vi "Extract Data.vi"(8 "error in (no error)":errorcluster caption="entrée d'erreur (pas d'erreur)", 11 "Parsing Data RADIO_ERP1 en entrée":refnum<class "Parsing Data RADIO_ERP1_D5.lvclass">) -> (0 "error out":errorcluster caption="sortie d'erreur", 3 "Parsing Data RADIO_ERP1 en sortie":refnum<class "Parsing Data RADIO_ERP1_D5.lvclass">)   [LabVIEW 2020, in "Library Instrument & Equipement.lvlib" / "Library UART.lvlib" / "Parsing Data RADIO_ERP1_D5.lvclass"]
uses:
  Parsing Data RADIO_ERP1_D5.lvclass
  C:/Users/ngarcin/OneDrive - Altyor/Standard TB/Class/UART/UART Enocean/Parsing Data Enocean (Default)/Parsing Data Enocean (Default).lvclass
  Parsing Data RADIO_ERP1_D5.lvclass/Parsing Data RADIO_ERP1_D5.ctl
  Commun VI/Library Commun.lvlib
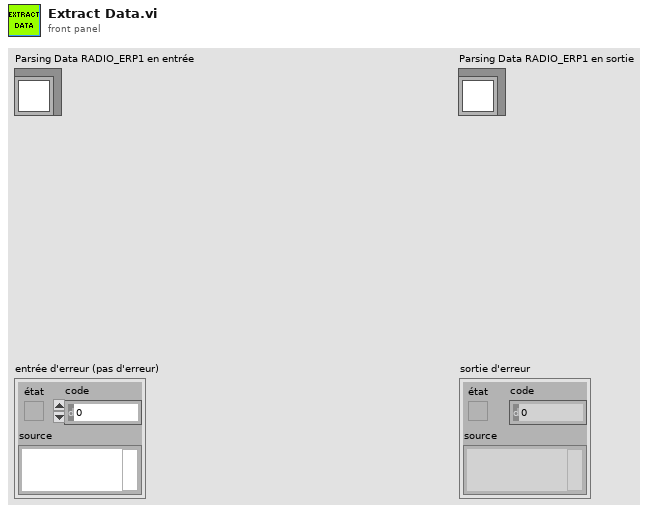
[diagram p1: front panel]
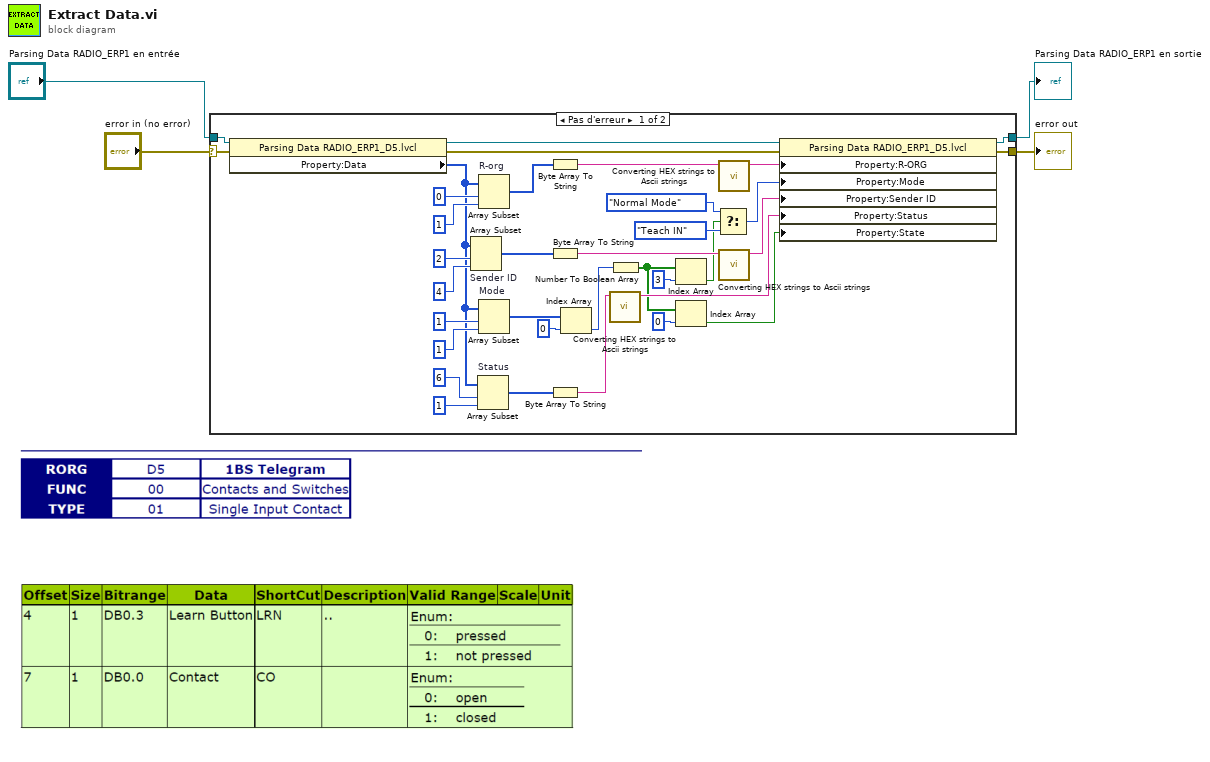
[diagram p0: block diagram]
diagram:
  n1 = case shown="Pas d'erreur" "error in (no error)" {
    selector: "error in (no error)" -> [w25 w41]
    tunnel: [w24 w41] -> w4
    tunnel: [w26 w40] -> w3
    tunnel: "Parsing Data RADIO_ERP1 en entrée" -> [w27 w40]
    frame No Error {
      n2 = property class="Parsing Data RADIO_ERP1_D5.lvcl"(reference=w27, error in=w25) -> (reference out=w39:refnum<class "Parsing Data RADIO_ERP1_D5.lvclass">, error out=w28:errorcluster, "Property:Data"=w15:u8[])
      n3 = Array Subset "Sender ID"(array=w15, index=2 ("indice"), length=4 ("longueur")) -> (w34:u8[])
      n4 = Array Subset "Status"(array=w15, index=6 ("indice"), length=1 ("indice")) -> (w29:u8[])
      n5 = Array Subset "R-org"(array=w15, index=0 ("indice"), length=1 ("longueur")) -> (w37:u8[])
      n6 = Array Subset "Mode"(array=w15, index=1 ("indice"), length=1 ("longueur")) -> (w13:u8[])
      n7 = Byte Array To String(unsigned byte array=w37) -> (string=w36:string)
      n8 = Byte Array To String(unsigned byte array=w34) -> (string=w33:string)
      n9 = Byte Array To String(unsigned byte array=w29) -> (string=w31:string)
      n10 = Index Array(array=w13, index=0 ("indice")) -> (element=w12:u8)
      n11 = call "Converting HEX strings to Ascii strings.vi"("chaîne IN"=w31) -> ("Chaîne OUT"=w30:string)  [unwired: 9 in, 1 out]
      n12 = Number To Boolean Array(number=w12) -> (Boolean array=w10:bool[])
      n13 = Index Array(array=w10, index=3 ("indice")) -> (element=w7:bool)
      n14 = Index Array(array=w10, index=0 ("indice")) -> (element=w9:bool)
      n15 = Select(t=enum16{"Teach IN", "Normal Mode"}."Normal Mode" ("cas vrai"), s=w7, f=enum16{"Teach IN", "Normal Mode"}."Teach IN" ("Mode")) -> (s? t:f=w6:enum16{"Teach IN", "Normal Mode"})
      n16 = call "Converting HEX strings to Ascii strings.vi"("chaîne IN"=w36) -> ("Chaîne OUT"=w35:string)  [unwired: 9 in, 1 out]
      n17 = call "Converting HEX strings to Ascii strings.vi"("chaîne IN"=w33) -> ("Chaîne OUT"=w32:string)  [unwired: 9 in, 1 out]
      n18 = property class="Parsing Data RADIO_ERP1_D5.lvcl"(reference=w39, error in=w28, "Property:R-ORG"=w35, "Property:Mode"=w6, "Property:Sender ID"=w32, "Property:Status"=w30, "Property:State"=w9) -> (reference out=w26:refnum<class "Parsing Data RADIO_ERP1_D5.lvclass">, error out=w24:errorcluster)
    }
    frame Error {
    }
  }
  "error out" <- w4
  "Parsing Data RADIO_ERP1 en sortie" <- w3
